vi "AndrewStruthers_StrainGageLab.vi"() -> ()   [LabVIEW 2018]
uses:
  <vilib>/express/express shared/transition.llb/Dynamic To Waveform Array.vi
  <vilib>/express/express arith-compare/Formula/Block/exnFormulaBlock how many pts in the wave.vi
  <vilib>/express/express shared/ex_Modify Signal Name.vi
  <vilib>/express/express shared/transition.llb/Waveform Array To Dynamic.vi
  <vilib>/express/express arith-compare/Formula/XNode/ExpressFormulaBlockNode.xnode
panel:
  in  "?":bool
  out "No Strain":bool
  out "Tension":bool
  out "Compression":bool
  out "Strain (e)":dbl
  out "Voltage (V)":dbl
  out "Strain":dynamicdata(graph)
  out "Voltage":dynamicdata(graph)
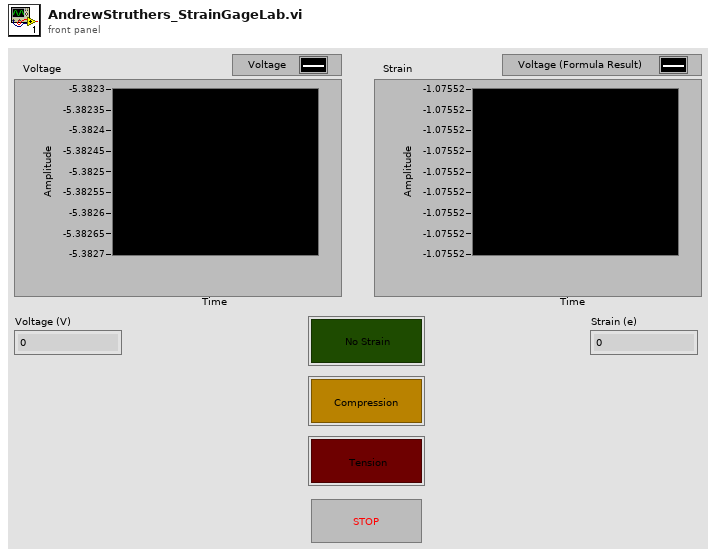
[diagram p1: front panel]
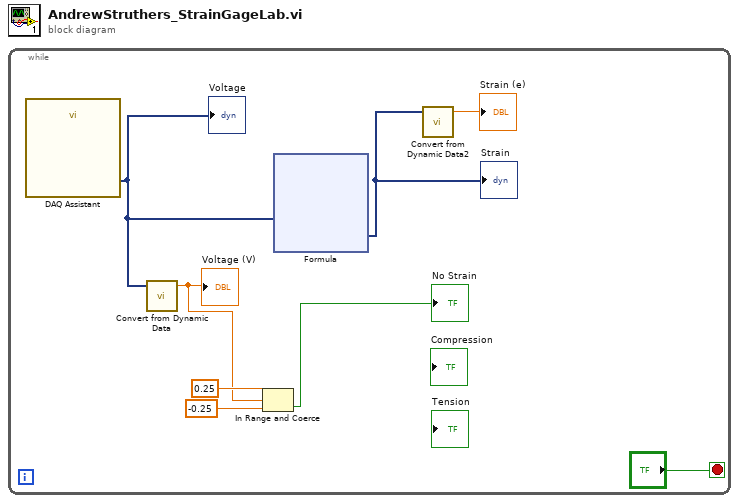
[diagram p0: block diagram]
diagram:
  n1 = while {
    stop <- "?" stop-if-true
    n2 = call "DAQ Assistant"() -> ("data"=w5:dynamicdata)  [unwired: 16 in, 3 out]
    "Voltage" <- w5
    n3 = call "Convert from Dynamic Data"("Dynamic Data Type"=w5) -> ("Scalar"=w2:dbl)  [unwired: 3 in]
    "Voltage (V)" <- w2
    n4 = In Range and Coerce(upper limit=0.25, x=w2, lower limit=-0.25) -> (In Range?=→"No Strain":bool)  [unwired: 1 out]
    n5 = xnode "Formula"("V"=w5) -> ("Result"=w7:dynamicdata)  [unwired: 1 in, 1 out]
    "Strain" <- w7
    n6 = call "Convert from Dynamic Data2"("Dynamic Data Type"=w7) -> ("Scalar"=→"Strain (e)":dbl)  [unwired: 3 in]
  }
